vi "Error - Log.vi"(8 "error in (no error)":errorcluster, 11 "Error Data":T1) -> (0 "error out":errorcluster)   [LabVIEW 2017]
doc: "Maintain an external Log file.\n[Covers: EH4]"
uses:
  Controls/Error Data.ctl
  Controls/Error Type.ctl
  Controls/Error Source.ctl
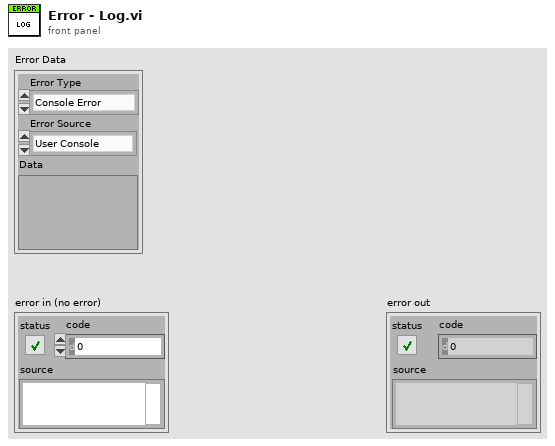
[diagram p1: front panel]
types:
  T1 = typedef "Error Data.ctl" = cluster{"Error Type":T2, "Error Source":T3, "Data":variant}
  T2 = typedef "Error Type.ctl" = enum16{"Console Error", "Sensor Interface IO Error", "Process Step Error"}
  T3 = typedef "Error Source.ctl" = enum16{"User Console", "Display Console", "Sensor Interface"}
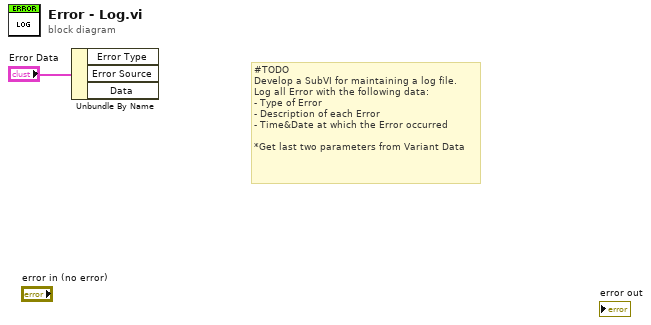
[diagram p0: block diagram]
diagram:
  # "#TODO\nDevelop a SubVI for maintaining a log file.\nLog all Error with the following data:\n- Type of Error\n- Description of each Error\n- Time&Date at which the Error occurred\n\n*Get last two parameters from Variant Data"
  n1 = Unbundle By Name("Error Data") -> ()  [unwired: 3 out]
